vi "Node Controller Stop.vi"(8 "error in (no error)":errorcluster, 11 "Node Controller in":refnum<class "Node Controller.lvclass">) -> (0 "error out":errorcluster, 3 "Node Controller out":refnum<class "Node Controller.lvclass">)   [LabVIEW 2024, in "Node Controller.lvclass"]
uses:
  Node Controller.lvclass
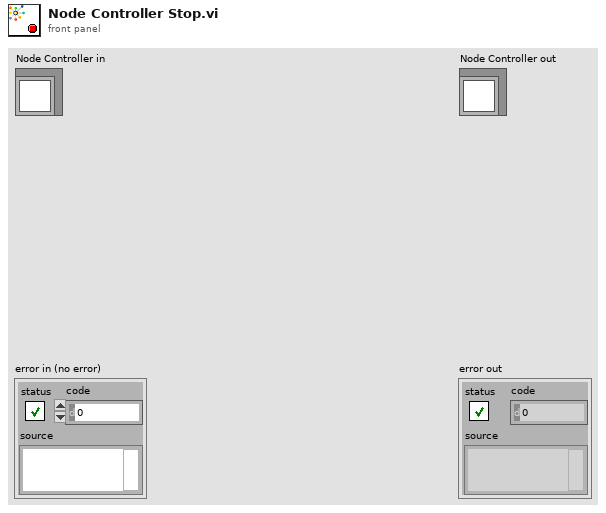
[diagram p1: front panel]
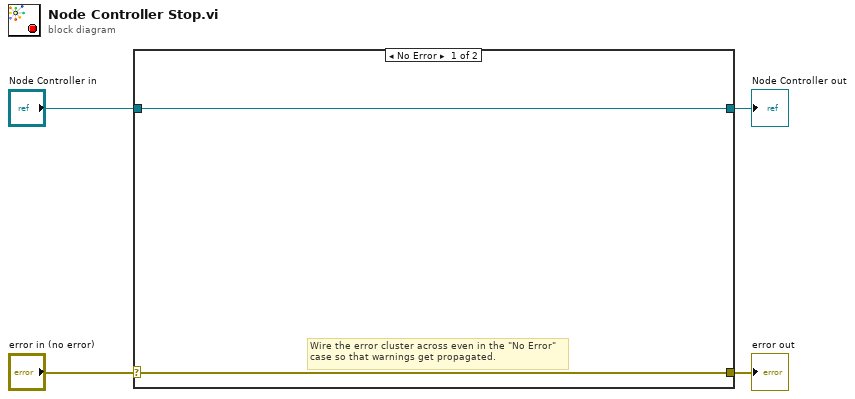
[diagram p0: block diagram]
diagram:
  n1 = case shown="No Error" "error in (no error)" {
    selector: "error in (no error)" -> [w5 w8]
    tunnel: [w5 w8] -> w3
    tunnel: [w6 w7] -> w1
    tunnel: "Node Controller in" -> [w6 w7]
    frame No Error {
      # "Wire the error cluster across even in the \"No Error\"\ncase so that warnings get propagated."
    }
    frame Error {
    }
  }
  "error out" <- w3
  "Node Controller out" <- w1
